vi "robot pause.vi"() -> ()   [LabVIEW 2020]
panel:
  in  "robot pause":bool
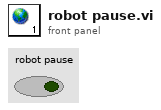
[diagram p1: front panel]
diagram:
